vi "VNum Info.vi"(8 "error in (no error)":errorcluster, 11 "Variant":variant) -> (0 "error out":errorcluster, 2 "# Bytes":u32, 3 "# Bits":u32, 4 "Fractional":bool=TRUE, 6 "Signed":bool, 7 "Complex":bool)   [LabVIEW 2020, in "LV Tiff.lvlib"]
uses:
  LV Tiff.lvlib
  <vilib>/Utility/Data Type/NI_Data Type.lvlib
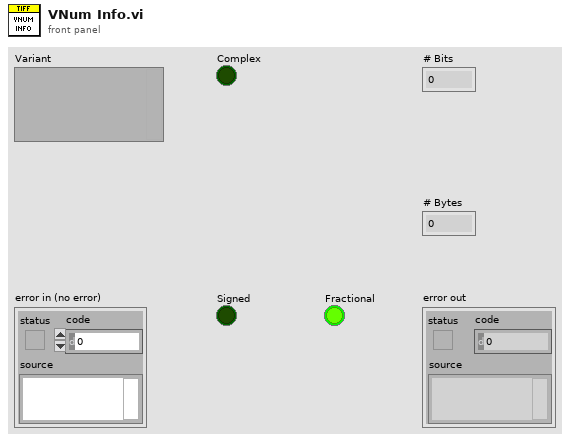
[diagram p1: front panel]
types:
  T1 = typedef "LVNumericRepresentation.ctl" = enum32{"Extended Precision", "Double Precision", "Single Precision", "Long", "Word", "Byte", "Unsigned Long", "Unsigned Word", "Unsigned Byte", "Complex Extended", "Complex Double", "Complex Single", "Quad", "Unsigned Quad", "Fixed-Point"}
  T2 = typedef "LVFixedPointRepBitsTypeDef.ctl" = cluster{"Signed":bool, "Word Length":u32, "Integer Word Length":i32}
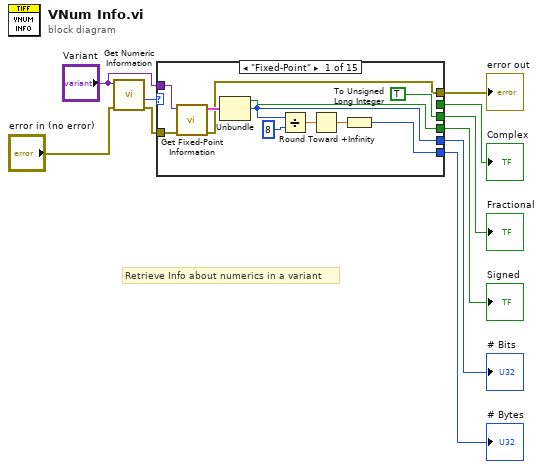
[diagram p0: block diagram]
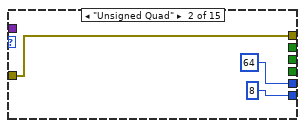
[diagram p2: hidden frame]
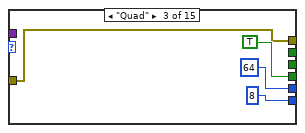
[diagram p3: hidden frame]
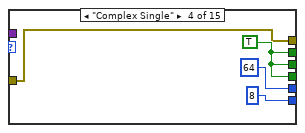
[diagram p4: hidden frame]
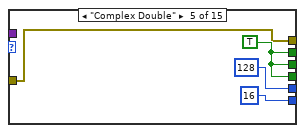
[diagram p5: hidden frame]
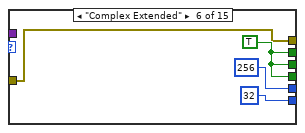
[diagram p6: hidden frame]
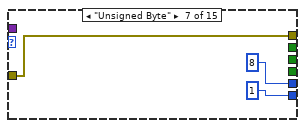
[diagram p7: hidden frame]
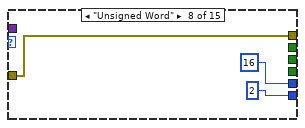
[diagram p8: hidden frame]
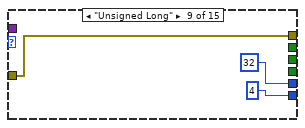
[diagram p9: hidden frame]
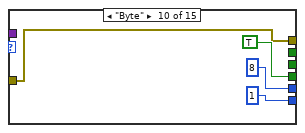
[diagram p10: hidden frame]
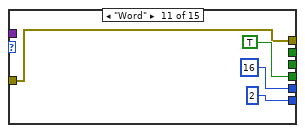
[diagram p11: hidden frame]
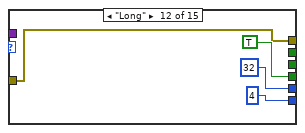
[diagram p12: hidden frame]
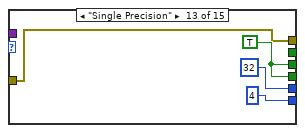
[diagram p13: hidden frame]
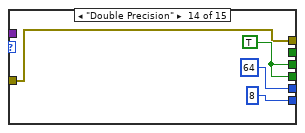
[diagram p14: hidden frame]
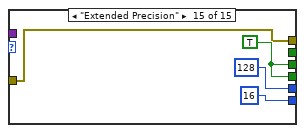
[diagram p15: hidden frame]
diagram:
  # "Retrieve Info about numerics in a variant"
  n1 = call <vilib>:"Get Numeric Information.vi"("error in (no error)"="error in (no error)", "variant"="Variant") -> ("error out"=w2:errorcluster, "representation"=w10:T1)  [unwired: 6 in, 2 out]
  n2 = case shown="\"Fixed-Point\"" w10 {
    tunnel: [TRUE _ _ w30 w34 w38 _ _ _ _ _ _ w63 w67 w71] -> w9
    tunnel: [w19 _ TRUE ("Signed") w30 w34 w38 _ _ _ TRUE ("Signed") TRUE ("Signed") TRUE ("Signed") w63 w67 w71] -> w8
    tunnel: "Variant" -> [w21 _ _ _ _ _ _ _ _ _ _ _ _ _ _]
    tunnel: [w17 u32 64 ("Word Length") u32 64 ("Word Length") u32 64 ("Word Length") u32 128 ("Word Length") u32 256 ("Word Length") u32 8 ("Word Length") u32 16 ("Word Length") u32 32 ("Word Length") u32 8 ("Word Length") u32 16 ("Word Length") u32 32 ("Word Length") u32 32 ("Word Length") u32 64 ("Word Length") u32 128 ("Word Length")] -> w6
    tunnel: [w13 u32 8 u32 8 u32 8 u32 16 u32 32 u32 1 u32 2 u32 4 u32 1 u32 2 u32 4 u32 4 u32 8 u32 16] -> w5
    tunnel: [_ _ _ w30 w34 w38 _ _ _ _ _ _ _ _ _] -> w4
    tunnel: w2 -> [w12 w22 w25 w29 w33 w37 w41 w44 w47 w50 w54 w58 w62 w66 w70]
    tunnel: [w11 w22 w25 w29 w33 w37 w41 w44 w47 w50 w54 w58 w62 w66 w70] -> w1
    frame "Fixed-Point" {
      n3 = call <vilib>:"Get Fixed-Point Information.vi"("error in (no error)"=w12, "variant"=w21) -> ("error out"=w11:errorcluster, "FXP representation"=w20:T2)  [unwired: 6 in, 2 out]
      n4 = Unbundle(w20) -> ("Signed"=w19:bool, "Word Length"=w17:u32)  [unwired: 1 out]
      n5 = Divide(x=w17, y=u32 8) -> (x/y=w15:dbl)
      n6 = Round Toward +Infinity(x=w15) -> (ceil(x): smallest int >= x=w14:dbl)
      n7 = To Unsigned Long Integer(number=w14) -> (unsigned 32bit integer=w13:u32)
    }
    frame "Unsigned Quad" {
    }
    frame "Quad" {
    }
    frame "Complex Single" {
      w30 = TRUE
    }
    frame "Complex Double" {
      w34 = TRUE
    }
    frame "Complex Extended" {
      w38 = TRUE
    }
    frame "Unsigned Byte" {
    }
    frame "Unsigned Word" {
    }
    frame "Unsigned Long" {
    }
    frame "Byte" {
    }
    frame "Word" {
    }
    frame "Long" {
    }
    frame "Single Precision" {
      w63 = TRUE
    }
    frame "Double Precision" {
      w67 = TRUE
    }
    frame "Extended Precision" {
      w71 = TRUE
    }
  }
  "Fractional" <- w9
  "Signed" <- w8
  "# Bits" <- w6
  "# Bytes" <- w5
  "Complex" <- w4
  "error out" <- w1
